vi "RunBook.vi"() -> ()   [LabVIEW 2012]
panel:
  out "Book?":bool
  # "Loading the book and starting the server..."
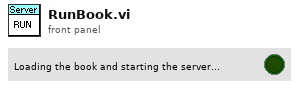
[diagram p1: front panel]
types:
  T1 = typedef "PathsGlobal.ctl" = cluster{"Root":path, "Shelves":path, "Cmds":path, "Plugins":path}
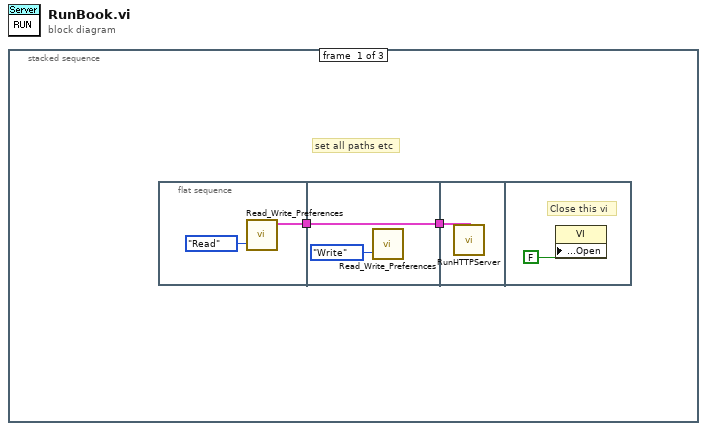
[diagram p0: block diagram]
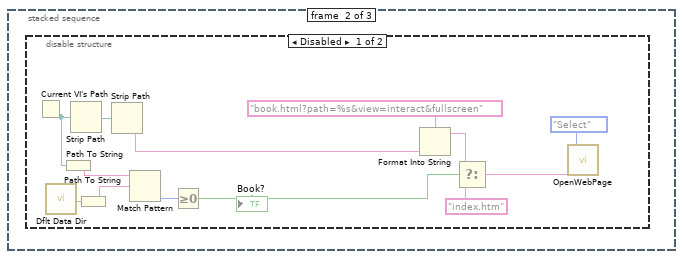
[diagram p2: hidden frame]
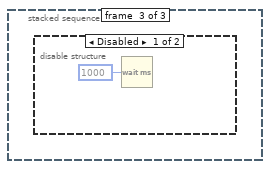
[diagram p4: hidden frame]
diagram:
  n1 = stacked-sequence {
    frame #0 {
      # "set all paths etc"
      n2 = flat-sequence {
        tunnel: [w3] -> w2
        tunnel: w2 -> [w5]
        tunnel: [w5] -> w1
        tunnel: w1 -> [w7]
        frame #0 {
          n3 = call <userlib>:"Read_Write_Preferences.vi"("task"=enum16{"Read", "Write"}."Read") -> ("Paths"=w3:T1)  [unwired: 4 out]
        }
        frame #1 {
          n4 = call <userlib>:"Read_Write_Preferences.vi"("task"=enum16{"Read", "Write"}."Write") -> ()  [unwired: 5 out]
        }
        frame #2 {
          n5 = call <userlib>:"RunHTTPServer.vi"("Paths"=w7) -> ()
        }
        frame #3 {
          # "Close this vi"
          n6 = property class="VI"("Front Panel Window:Open"=FALSE) -> ()  [unwired: 2 in, 2 out]
        }
      }
    }
    frame #1 {
      n7 = disable-structure shown="Disabled" {
        frame Disabled {
          n8 = Current VI's Path() -> (path=w16:path)
          n9 = call <vilib>:"Dflt Data Dir.vi"() -> ("App:Default Data Directory"=w15:path)
          n10 = Path To String(path=w16) -> (string=w14:string)
          n11 = Strip Path(path=w16) -> (stripped path=w20:path)  [unwired: 1 out]
          n12 = Path To String(path=w15) -> (string=w13:string)
          n13 = Strip Path(path=w20) -> (name=w19:string)  [unwired: 1 out]
          n14 = Match Pattern(string=w14, regular expression=w13) -> (offset past match=w12:i32)  [unwired: 4 out]
          n15 = Greater Or Equal To 0?(x=w12) -> (x >= 0?=w11:bool)
          "Book?" <- w11
          n16 = Format Into String(format string="book.html?path=%s&view=interact&fullscreen", w19) -> (resulting string=w18:string)  [unwired: 2 in, 1 out]
          n17 = Select(t=w18, s=w11, f="index.htm" ("format string")) -> (s? t:f=w9:string)
          n18 = call <userlib>:"OpenWebPage.vi"("Path"=w9, "WebPage"=enum16{"Shelves", "About", "Select", "Generic"}."Select") -> ()  [unwired: 2 out]
        }
        frame Enabled {
        }
      }
    }
    frame #2 {
      n19 = disable-structure shown="Disabled" {
        frame Disabled {
          n20 = Wait (ms)(milliseconds to wait=u32 1000) -> ()  [unwired: 1 out]
        }
        frame Enabled {
        }
      }
    }
  }
